vi "Initialise Command Reader.vi"(8 "error in (no error)":errorcluster) -> (0 "error out":errorcluster, 3 "Refnum out":refnum<k21>)   [LabVIEW 2017]
uses:
  HostRTCommunication/Command and Parameters.ctl
  HostRTCommunication/Commands.ctl
  <vilib>/dex/Stream Element Allocation Mode.ctl
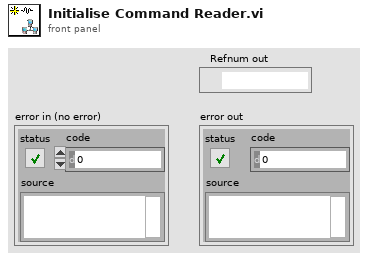
[diagram p1: front panel]
types:
  T1 = typedef "Stream Element Allocation Mode.ctl" = u32
  T2 = typedef "Command and Parameters.ctl" = cluster{"Command":T3, "Command Parameters":variant[]}
  T3 = typedef "Commands.ctl" = enum16{"Set Center Frequency", "Set AGC State", "Set Number Of Averages", "Set Tuner Gain Mode", "Set Frequency Correction", "Set Sample Rate", "Set Manual Gain Value"}
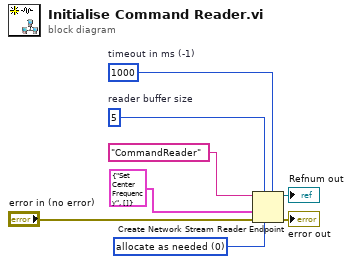
[diagram p0: block diagram]
diagram:
  w6 = 1000  # timeout in ms (-1)
  w5 = 5  # reader buffer size
  w4 = T1 0 items=["allocate as needed", "pre-allocate"] ("element allocation mode")
  n1 = Create Network Stream Reader Endpoint(5:w6, 6:w4, 7:w5, 8:"error in (no error)", 9:T2 {"Command"=enum."Set Center Frequency", "Command Parameters"=[]}, 11:"CommandReader" ("reader name")) -> (0:→"error out":errorcluster, 3:→"Refnum out":refnum<k21>)  [unwired: 1 in]
